vi "createEnumeration.vi"(8 "error in (no error)":errorcluster, 11 "Module in":refnum<class "Module.lvclass">) -> (0 "error out":errorcluster, 3 "Module out":refnum<class "Module.lvclass">)   [LabVIEW 2016, in "Module.lvclass"]
uses:
  Module.lvclass
  Enumeration/Enumeration.lvclass
  Module.lvclass/Module.ctl
  Enumeration/Enumeration.lvclass/Enumeration.ctl
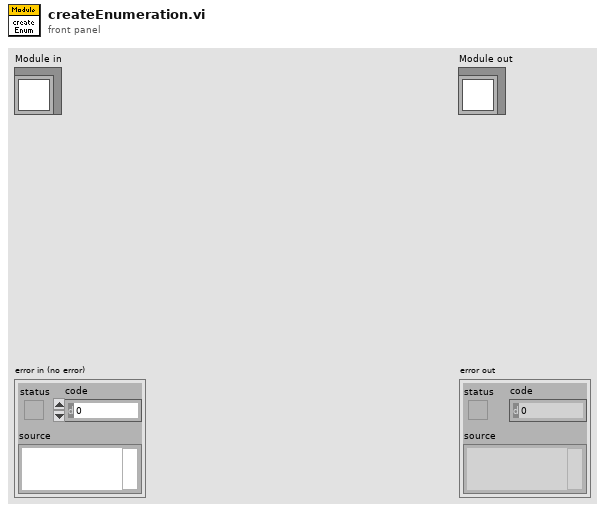
[diagram p1: front panel]
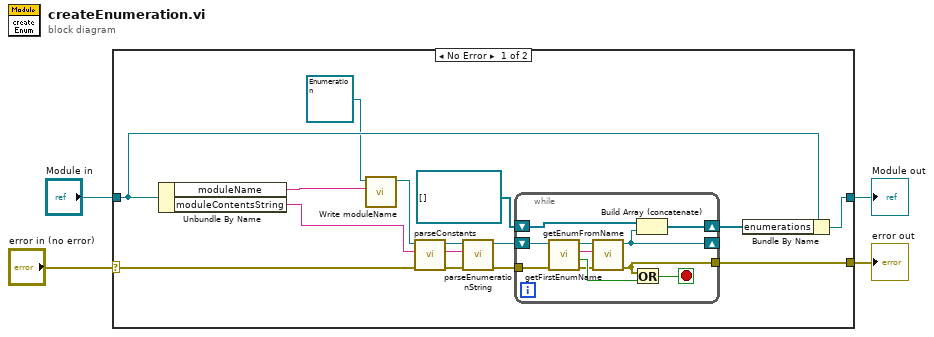
[diagram p0: block diagram]
diagram:
  n1 = case shown="No Error" "error in (no error)" {
    selector: "error in (no error)" -> [w14 w32]
    tunnel: [w6 w32] -> w3
    tunnel: [w19 w31] -> w1
    tunnel: "Module in" -> [w16 w31]
    frame No Error {
      n2 = Unbundle By Name(w16) -> ("moduleName"=w15:string, "moduleContentsString"=w9:string)
      n3 = call "Write moduleName.vi"("moduleName"=w15, "Enumeration in"=refnum<class "Enumeration.lvclass"> refnum ("Enumeration.lvclass")) -> ("Enumeration out"=w12:refnum<class "Enumeration.lvclass">)  [unwired: 8 in, 1 out]
      n4 = call "parseConstants.vi"("error in (no error)"=w14, "IDLString"=w9, "Enumeration in"=w12) -> ("error out"=w13:errorcluster, "IDLConstants"=w5:string, "Enumeration out"=w11:refnum<class "Enumeration.lvclass">)  [unwired: 6 in]
      n5 = call "parseEnumerationString.vi"("error in (no error)"=w13, "IDLConstants"=w5, "Enumeration in"=w11) -> ("error out"=w7:errorcluster, "Enumeration out"=w8:refnum<class "Enumeration.lvclass">)  [unwired: 7 in]
      n6 = while {
        shift-right: [w29] -> w17
        shift-left: refnum<class "Enumeration.lvclass">[] [] ("enumerations") -> [w30]
        tunnel: w7 -> [w28]
        tunnel: [w21] -> w6
        shift-right: [w20] -> _
        shift-left: w8 -> [w27]
        stop <- w26 stop-if-true
        n7 = call "getFirstEnumName.vi"("error in (no error)"=w28, "Enumeration in"=w27) -> ("error out"=w24:errorcluster, "enumListIsEmpty"=w25:bool, "FirstEnumName"=w23:string, "Enumeration out"=w22:refnum<class "Enumeration.lvclass">)  [unwired: 6 in]
        n8 = call "getEnumFromName.vi"("error in (no error)"=w24, "name"=w23, "Enumeration in"=w22) -> ("error out"=w21:errorcluster, "Enumeration out"=w20:refnum<class "Enumeration.lvclass">)  [unwired: 7 in]
        n9 = Or(x=w21, y=w25) -> (x .or. y?=w26:bool)
        n10 = Build Array (concatenate)(w30, w20) -> (w29:refnum<class "Enumeration.lvclass">[])
      }
      n11 = Bundle By Name(cluster=w16, "enumerations"=w17) -> (w19:refnum<class "Module.lvclass">)
    }
    frame Error {
    }
  }
  "error out" <- w3
  "Module out" <- w1
